vi "testStringIncluded.vi"() -> ()   [LabVIEW 2019, in "AssertionTest.lvlib" / "ErrorMessageContainsString.lvlib"]
uses:
  ErrorMessageContainsString.lvlib
  Assertion/Assertion.lvlib
  <vilib>/Utility/error.llb/Error Cluster From Error Code.vi
  <vilib>/ErrorRing/Error Ring.xnode
panel:
  out "error out":errorcluster
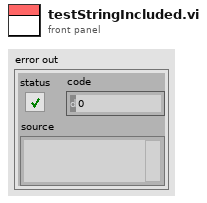
[diagram p1: front panel]
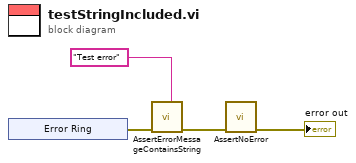
[diagram p0: block diagram]
diagram:
  n1 = xnode "Error Ring"() -> ("error out"=w3:errorcluster)
  n2 = call "AssertErrorMessageContainsString.vi"("Expected"="Test error", "error in (no error)"=w3) -> ("error out"=w2:errorcluster)  [unwired: 9 in]
  n3 = call "AssertNoError.vi"("error in (no error)"=w2) -> ("error out"=→"error out":errorcluster)  [unwired: 10 in]
